vi "ziExample-Module-PIDAdvisor.vi"() -> ()   [LabVIEW 2009]
doc: "Control a Zurich instrument device via the LabOne Labview API. \nRequirements: Zurich Instruments HF2 +MF or UHFLI +MF \nPlease connect Signal input 1 and Signall Output 1.\nThis example shows how to configure a PID to regulate the output amplitude in order to achieve a constant input amplitude.\nThis example suggests a PID configuration via the PID advisor.\n\n© Zurich Instruments AG, www.zhinst.com"
uses:
  <instrlib>/Zurich Instruments LabOne/Public/ziTypeHandle.ctl
  <instrlib>/Zurich Instruments LabOne/Public/Modules/ziTypeModEnum.ctl
  <instrlib>/Zurich Instruments LabOne/Public/Modules/ziModSetValueBinary.vi
  <instrlib>/Zurich Instruments LabOne/Public/Configure/ziSetValueDouble.vi
  <instrlib>/Zurich Instruments LabOne/Public/Configure/ziSetValueDoubleArray.vi
  <instrlib>/Zurich Instruments LabOne/Public/Configure/ziGetValueString.vi
  <instrlib>/Zurich Instruments LabOne/Public/Modules/ziModSetValueDouble.vi
  <instrlib>/Zurich Instruments LabOne/Public/Modules/ziModSetValueDoubleArray.vi
  <instrlib>/Zurich Instruments LabOne/Public/Modules/ziModGetDoubleData.vi
  <instrlib>/Zurich Instruments LabOne/Public/Modules/ziModGetAdvisorData.vi
  <instrlib>/Zurich Instruments LabOne/Zurich Instruments LabOne.lvlib
panel:
  out "VALUE":dbl(graph)
  out "PID SHIFT":dbl(graph)
  out "demod/timeconstant":dbl
  out "Error Out":errorcluster
  out "Handle Out":T1 {"Handle" format="0x%08x"; "Conn" format="0x%08x"}
  in  "Calculate":bool
  in  "stop":bool
  out "PID ERROR":dbl(graph)
  in  "Address":string="DEV"
  in  "bw":dbl=100.0 caption="target BW (Hz)"
  in  "Mode":dbl(ring)=3.0 items=["P"=1.0, "I"=2.0, "PI"=3.0, "PID"=7.0, "PIDF"=15.0]
  out "i":dbl caption="I"
  out "p":dbl caption="P"
  out "dlimittimeconstant":dbl
  out "rate":dbl caption="Rate (Hz)"
  out "d":dbl caption="D"
  out "Step Response":cluster{"grid":dbl[], "r_avg":dbl[]}(graph)
  out "Bode Gain":cluster{"grid":dbl[], "r_avg":dbl[]}(graph)
  out "Bode Phase":cluster{"grid":dbl[], "r_avg":dbl[]}(graph)
  out "Selected Device":string
  in  "subscribepath":string="pidAdvisor/*" caption="Subscribe Path"
  # "ziExample-SweepModul.vi\nRequirements: UHFLI, HF2, MFLI +PID\nsee block diagram for VI description"
  # "Tested Devices:\n- UHFLI+PID \n- HF2+PID\n- MFLI+PID"
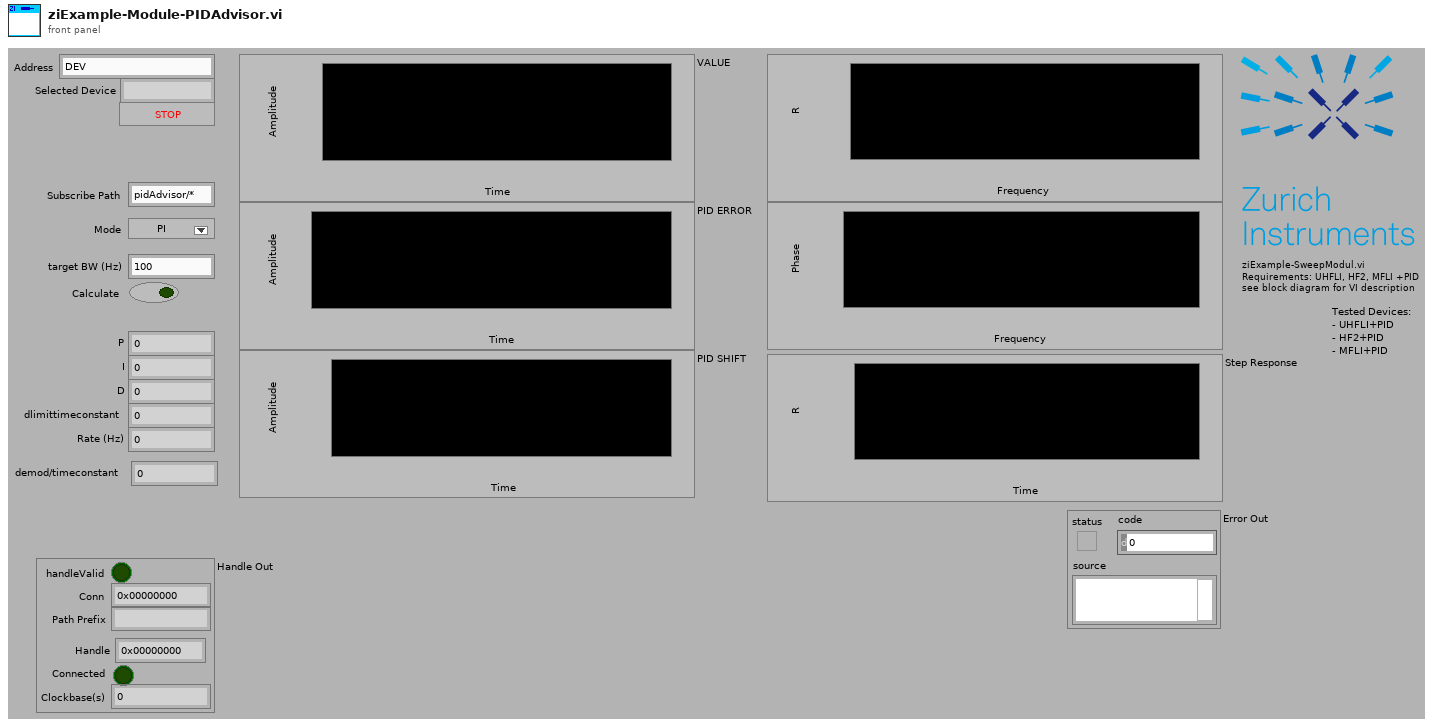
[diagram p1: front panel]
types:
  T1 = typedef "Zurich Instruments LabOne.lvlib/ziTypeHandle.ctl" = cluster{"handleValid":bool, "Conn":u64, "Path Prefix":string, "Handle":u64, "Connected":bool, "Clockbase(s)":dbl}
  T2 = typedef "Zurich Instruments LabOne.lvlib/ziTypeModEnum.ctl" = u16
  T3 = typedef "Zurich Instruments LabOne.lvlib/ziTypeModHandle.ctl" = cluster{"handleValid":bool, "Conn":u64, "ModHandle":u64, "moduleID":string, "Path Prefix":string}
  T4 = typedef "Zurich Instruments LabOne.lvlib/ziTypeModResults.ctl" = cluster{"PathArray":string[], "ValueType":T5, "NoOfResults":u64, "ziGenericHeader":T6[]}
  T5 = typedef "Zurich Instruments LabOne.lvlib/ziTypePollType.ctl" = enum16{"NONE", "DOUBLE_DATA", "INTEGER_DATA", "DEMOD_SAMPLE", "SCOPE_WAVE_HF2", "AUXIN_SAMPLE", "DIO_SAMPLE", "BYTE_ARRAY", "PWA_WAVE", "9", "10", "11", "12", "13", "14", "15", "TREE_CHANGE_DEPRI", "17", "ERROR", "19", "20", "21", "22", "23", "24", "25", "26", "27", "28", "29", "30", "31", "DOUBLE_DATA_TS", "INTEGER_DATA_TS", "34", "SCOPE_WAVE", "SCOPE_WAVE_EX", "37", "BYTE_ARRAY_TS", "39", "40", "41", "42", "43", "44", "45", "CNT_DATA", "47", "TREE_CHANGE", "49", "50", "51", "52", "53", "54", "55", "56", "57", "58", "59", "60", "61", "62", "63", "SWEEPER_DATA", "SPECTRUM_DATA", "ADVISOR_DATA", "VECTOR_DATA", "IMP_DATA"}
  T6 = typedef "Zurich Instruments LabOne.lvlib/ziTypeModGenericHeader.ctl" = cluster{"HeaderType":enum8{"HEADER_TYPE_NONE", "HEADER_TYPE_SWTRIGGER", "HEADER_TYPE_SWEEPER"}, "SampleFormat":u8, "SystemTime":timestamp, "CreatedTimeStamp":u64, "ChangedTimeStamp":u64, "Flags":u32, "ChunkSizeBytes":u64, "Name":string, "Status":u32, "GroupIndex":u32, "Color":u32, "ActiveRow":u32, "TriggerNumber":u64, "GridRows":u32, "GridCols":u32, "GridMode":u32, "GridOperation":u32, "GridDirection":u32, "GridRepetitions":u32, "GridColDelta":dbl, "GridColOffset":dbl, "GridRowDelta":dbl, "GridRowOffset":dbl, "Bandwidth":dbl, "Center":dbl, "Nenbw":dbl}
  T7 = typedef "Zurich Instruments LabOne.lvlib/ziTypeModAdvisorWave.ctl" = cluster{"timestamp":u64, "sampleCount":u64, "flags":u8, "sampleFormat":u8, "grid":dbl[], "x":dbl[], "y":dbl[]}
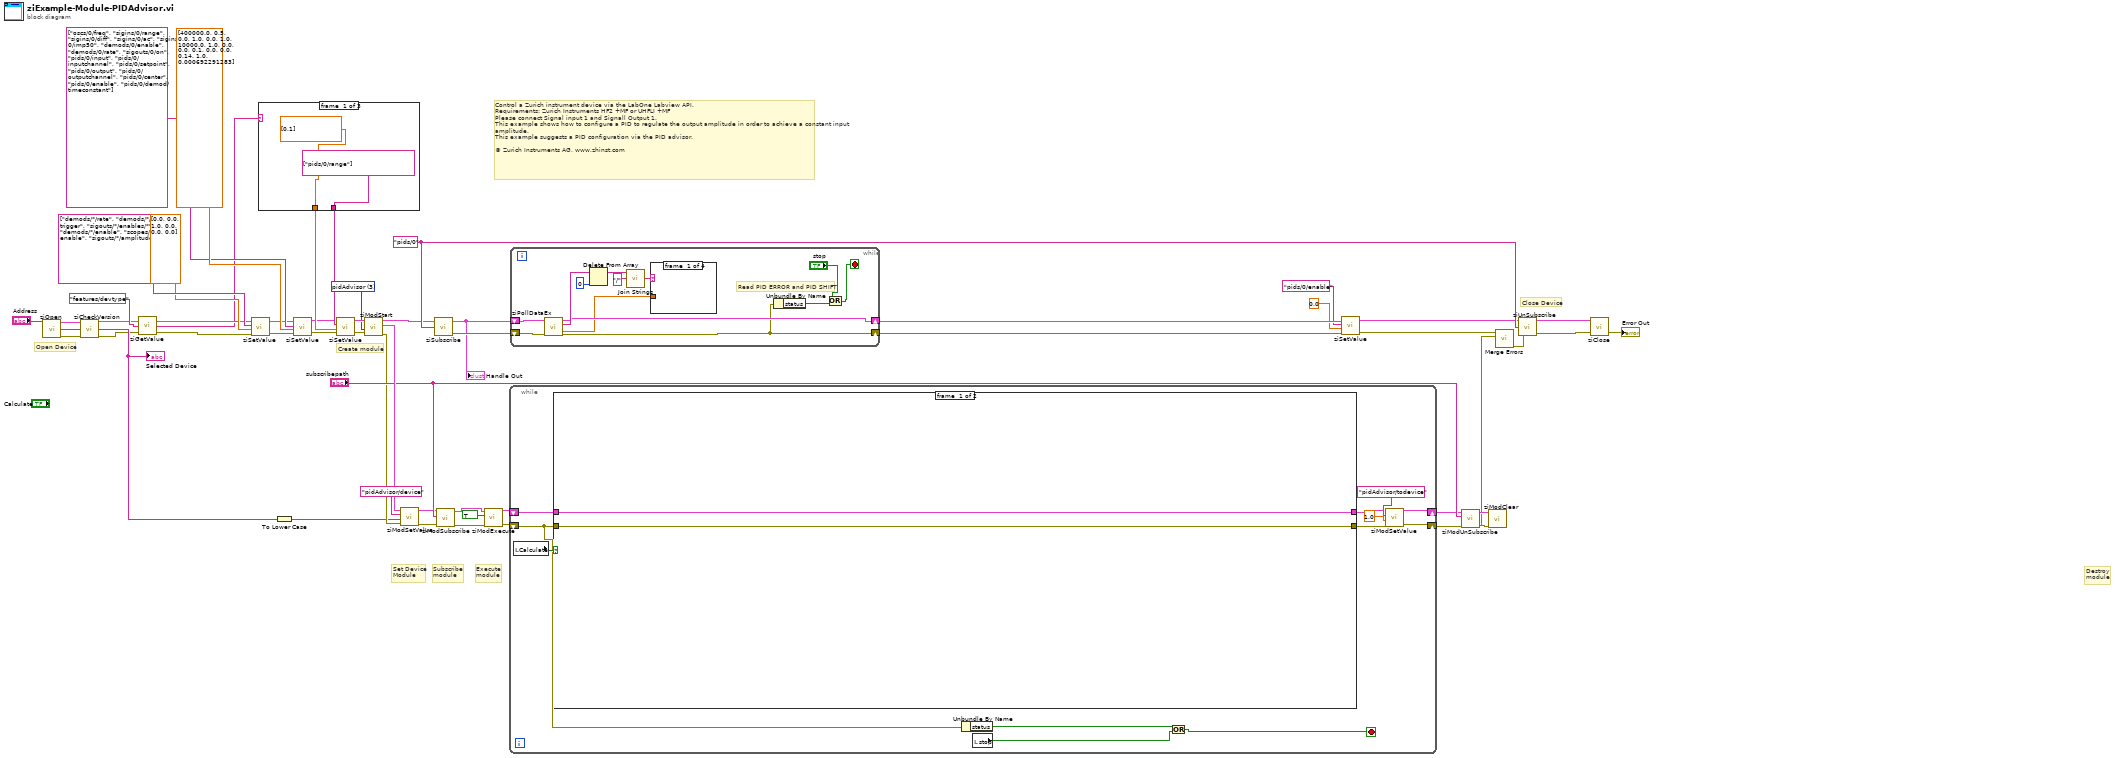
[diagram p0: block diagram]
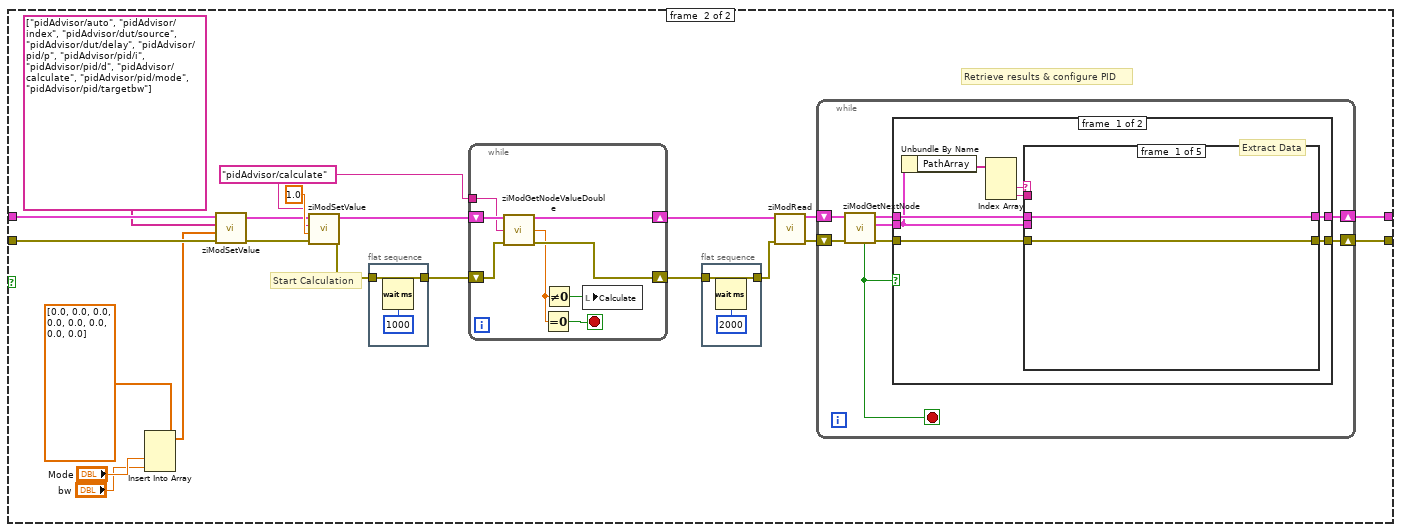
[diagram p2: hidden frame]
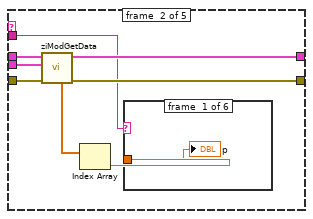
[diagram p3: hidden frame]
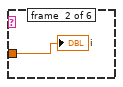
[diagram p4: hidden frame]
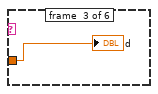
[diagram p5: hidden frame]
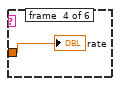
[diagram p6: hidden frame]
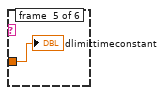
[diagram p7: hidden frame]
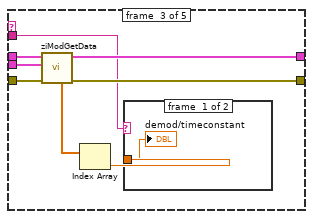
[diagram p9: hidden frame]
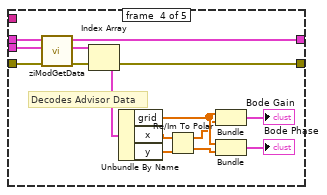
[diagram p11: hidden frame]
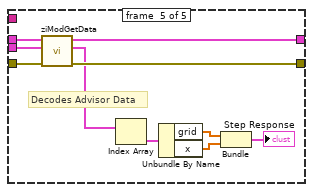
[diagram p12: hidden frame]
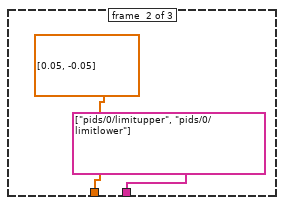
[diagram p14: hidden frame]
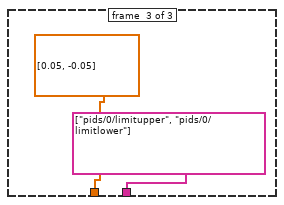
[diagram p15: hidden frame]
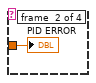
[diagram p16: hidden frame]
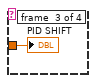
[diagram p17: hidden frame]
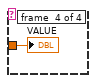
[diagram p18: hidden frame]
diagram:
  w1 = T2 3 items=["sweep", "scopeModule", "dataAcquisitionModule", "pidAdvisor", "awgModule", "impedanceModule", "multiDeviceSyncModule", "zoomFFT", "trigger", "deviceSettings", "record"] ("module Id")
  w29 = "pids/0" ("Path ()")
  # "Control a Zurich instrument device via the LabOne Labview API. \nRequirements: Zurich Instruments HF2 +MF or UHFLI +MF \nPlease connect Signal input 1 and Signall Output 1.\nThis example shows how to configure a PID to regulate the output amplitude in order to achieve a constant input amplitude.\nThis example suggests a PID configuration via the PID advisor.\n\n© Zurich Instruments AG, www.zhinst.com"
  # "Execute\nmodule"
  # "Set Device\nModule"
  # "Subscribe\nmodule"
  # "Destroy\nmodule"
  # "Create module"
  # "Close Device"
  # "Open Device"
  n1 = call <instrlib>:"ziOpen.vi"("Address"="Address") -> ("Error Out"=w2:errorcluster, "Selected Device"=w27:string, "HandleOut"=w5:T1)  [unwired: 1 in, 2 out]
  "Selected Device" <- w27
  n2 = call <instrlib>:"ziCheckVersion.vi"("Handle In"=w5, "Error In"=w2) -> ("Handle Out"=w4:T1, "Error Out"=w3:errorcluster)  [unwired: 11 in, 1 out]
  n3 = call-poly <instrlib>:"ziGetValue.vi"("error in"=w3, "Path"="features/devtype", "Handle In"=w4) -> ("error out"=w8:errorcluster, "Value"=w6:string, "Handle Out"=w9:T1)
  n4 = call-poly <instrlib>:"ziSetValue.vi"("Error In"=w8, "Values"=dbl[] [0.0, 0.0, 1.0, 0.0, 0.0, 0.0], "Paths"=string[] ["demods/*/rate", "demods/*/trigger", "sigouts/*/enables/*", "demods/*/enable", "scopes/*/enable", "sigouts/*/amplitudes/*"], "Handle In"=w9) -> ("Error Out"=w10:errorcluster, "Handle Out"=w11:T1)  [unwired: 1 in]
  n5 = case shown="\"MFIA\", \"MFLI\"" w6 {
    tunnel: [dbl[] [0.1] dbl[] [0.05, -0.05] dbl[] [0.05, -0.05]] -> w34
    tunnel: [string[] ["pids/0/range"] string[] ["pids/0/limitupper", "pids/0/limitlower"] string[] ["pids/0/limitupper", "pids/0/limitlower"]] -> w33
    frame #0 {
    }
    frame #1 {
    }
    frame #2 {
    }
  }
  n6 = To Lower Case(string=w27) -> (all lower case string=w26:string)
  n7 = call-poly <instrlib>:"ziSetValue.vi"("Error In"=w10, "Values"=dbl[] [400000.0, 0.5, 0.0, 1.0, 0.0, 1.0, 10000.0, 1.0, 0.0, 0.0, 0.1, 0.0, 0.0, 0.14, 1.0, 0.000692291283], "Paths"=string[] ["oscs/0/freq", "sigins/0/range", "sigins/0/diff", "sigins/0/ac", "sigins/0/imp50", "demods/0/enable", "demods/0/rate", "sigouts/0/on", "pids/0/input", "pids/0/inputchannel", "pids/0/setpoint", "pids/0/output", "pids/0/outputchannel", "pids/0/center", "pids/0/enable", "pids/0/demod/timeconstant"], "Handle In"=w11) -> ("Error Out"=w18:errorcluster, "Handle Out"=w19:T1)  [unwired: 1 in]
  n8 = call-poly <instrlib>:"ziSetValue.vi"("Error In"=w18, "Values"=w34, "Paths"=w33, "Handle In"=w19) -> ("Error Out"=w53:errorcluster, "Handle Out"=w54:T1)  [unwired: 1 in]
  n9 = call <instrlib>:"ziModStart.vi"("Error In"=w53, "module Id"=w1, "Handle In"=w54) -> ("Error Out"=w37:errorcluster, "ModHandle Out"=w50:T3, "Handle Out"=w7:T1)  [unwired: 6 in]
  n10 = call-poly <instrlib>:"ziModSetValue.vi"("Error In"=w37, "Data"=w26, "Path"="pidAdvisor/device", "ModHandle In"=w50) -> ("Error Out"=w41:errorcluster, "ModHandle Out"=w40:T3)  [unwired: 6 in]
  n11 = call <instrlib>:"ziSubscribe.vi"("Path ()"=w29, "Handle In"=w7) -> ("error out"=w51:errorcluster, "Handle Out"=w38:T1)  [unwired: 2 in]
  "Handle Out" <- w38
  n12 = call <instrlib>:"ziModSubscribe.vi"("Error In"=w41, "Path"="subscribepath", "ModHandle In"=w40) -> ("Error Out"=w48:errorcluster, "ModHandle Out"=w47:T3)  [unwired: 6 in]
  n13 = call <instrlib>:"ziModExecute.vi"("Error In"=w48, "Modal (F)"=TRUE ("Modal"), "ziModHandle In"=w47) -> ("Error Out"=w49:errorcluster, "ziModHandle Out"=w39:T3)  [unwired: 5 in, 1 out]
  n14 = while {
    shift-right: [w67] -> w13
    shift-left: w39 -> [w72]
    shift-right: [w66] -> w12
    shift-left: w49 -> [w64]
    stop <- w61 stop-if-true
    n15 = local read "Calculate"() -> (w71:bool)
    n16 = case shown="True" w71 {
      tunnel: w72 -> [w73 w89]
      tunnel: w64 -> [w74 w90]
      tunnel: [w74 w82] -> w65
      tunnel: [w73 w83] -> w68
      frame #0 {
      }
      frame #1 {
        w76 = "pidAdvisor/calculate" ("Path")
        # "Extract Data"
        # "Retrieve results & configure PID"
        # "Start Calculation"
        n17 = Insert Into Array(array=dbl[] [0.0, 0.0, 0.0, 0.0, 0.0, 0.0, 0.0, 0.0], new element #1="Mode", new element #2="bw") -> (w77:dbl[])  [unwired: 1 in]
        n18 = call-poly <instrlib>:"ziModSetValue.vi"("Error In"=w90, "Values"=w77, "Paths"=string[] ["pidAdvisor/auto", "pidAdvisor/index", "pidAdvisor/dut/source", "pidAdvisor/dut/delay", "pidAdvisor/pid/p", "pidAdvisor/pid/i", "pidAdvisor/pid/d", "pidAdvisor/calculate", "pidAdvisor/pid/mode", "pidAdvisor/pid/targetbw"], "ModHandle In"=w89) -> ("Error Out"=w75:errorcluster, "ModHandle Out"=w78:T3)  [unwired: 6 in]
        n19 = call-poly <instrlib>:"ziModSetValue.vi"("Error In"=w75, "Value"=1.0, "Path"=w76, "ModHandle In"=w78) -> ("Error Out"=w88:errorcluster, "ModHandle Out"=w93:T3)  [unwired: 6 in]
        n20 = flat-sequence {
          tunnel: [w99] -> w87
          tunnel: w88 -> [w99]
          frame #0 {
            n21 = Wait (ms)(milliseconds to wait=u32 1000) -> ()  [unwired: 1 out]
          }
        }
        n22 = while {
          shift-right: [w169] -> w94
          shift-left: w93 -> [w172]
          shift-right: [w170] -> w85
          shift-left: w87 -> [w173]
          tunnel: w76 -> [w171]
          stop <- w168 stop-if-true
          n23 = call <instrlib>:"ziModGetNodeValueDouble.vi"("ModHandle In"=w172, "Path"=w171, "error in"=w173) -> ("ModHandle Out"=w169:T3, "Value"=w166:dbl, "error out"=w170:errorcluster)  [unwired: 10 in]
          n24 = Equal To 0?(x=w166) -> (x = 0?=w168:bool)
          n25 = Not Equal To 0?(x=w166) -> (x != 0?=w167:bool)
          n26 = local write "Calculate"(w167) -> ()
        }
        n27 = flat-sequence {
          tunnel: w85 -> [w96]
          tunnel: [w96] -> w84
          frame #0 {
            n28 = Wait (ms)(milliseconds to wait=u32 2000) -> ()  [unwired: 1 out]
          }
        }
        n29 = call <instrlib>:"ziModRead.vi"("error in"=w84, "ziModHandle In"=w94) -> ("error out"=w91:errorcluster, "ziModHandle Out"=w92:T3)  [unwired: 8 in]
        n30 = while {
          shift-right: [w101] -> w83
          shift-left: w92 -> [w106]
          shift-right: [w100] -> w82
          shift-left: w91 -> [w107]
          stop <- w102 stop-if-true
          n31 = call <instrlib>:"ziModGetNextNode.vi"("Error In"=w107, "ModHandle In"=w106) -> ("Error Out"=w104:errorcluster, "ModResults"=w103:T4, "ModHandle Out"=w105:T3, "NoData"=w102:bool)  [unwired: 6 in]
          n32 = case shown="False" w102 {
            tunnel: w105 -> [w115 w165]
            tunnel: w104 -> [w114 w164]
            tunnel: w103 -> [w111 _]
            tunnel: [w113 w165] -> w101
            tunnel: [w112 w164] -> w100
            frame #0 {
              n33 = Unbundle By Name(w111) -> ("PathArray"=w110:string[])
              n34 = Index Array(array=w110) -> (element #2=w108:string, element #3=w109:string)  [unwired: 3 in, 1 out]
              n35 = case shown="Default" w108 {
                tunnel: w115 -> [w117 w125 w138 w152 w162]
                tunnel: w111 -> [_ w124 w137 w153 w163]
                tunnel: w114 -> [w116 w123 w136 w151 w161]
                tunnel: [w116 w120 w133 w150 w160] -> w112
                tunnel: [w117 w122 w135 w149 w159] -> w113
                tunnel: w109 -> [_ w119 w132 _ _]
                frame #0 {
                }
                frame #1 {
                  n36 = call-poly <instrlib>:"ziModGetData.vi"("Error In"=w123, "ModResults"=w124, "ModHandle In"=w125) -> ("Error Out"=w120:errorcluster, "ModHandle Out"=w122:T3, "Value"=w118:dbl[])  [unwired: 4 in, 2 out]
                  n37 = Index Array(array=w118) -> (element=w121:dbl)  [unwired: 1 in]
                  n38 = case shown="\"d\"" w119 {
                    tunnel: w121 -> [w126 w127 w128 w129 w130 _]
                    frame #0 {
                      "p" <- w126
                    }
                    frame #1 {
                      "i" <- w127
                    }
                    frame #2 {
                      "d" <- w128
                    }
                    frame #3 {
                      "rate" <- w129
                    }
                    frame #4 {
                      "dlimittimeconstant" <- w130
                    }
                    frame #5 {
                    }
                  }
                }
                frame #2 {
                  n39 = call-poly <instrlib>:"ziModGetData.vi"("Error In"=w136, "ModResults"=w137, "ModHandle In"=w138) -> ("Error Out"=w133:errorcluster, "ModHandle Out"=w135:T3, "Value"=w131:dbl[])  [unwired: 4 in, 2 out]
                  n40 = Index Array(array=w131) -> (element=w134:dbl)  [unwired: 1 in]
                  n41 = case shown="\"timeconstant\"" w132 {
                    tunnel: w134 -> [w139 _]
                    frame #0 {
                      "demod/timeconstant" <- w139
                    }
                    frame #1 {
                    }
                  }
                }
                frame #3 {
                  # "Decodes Advisor Data"
                  n42 = call-poly <instrlib>:"ziModGetData.vi"("Error In"=w151, "ModResults"=w153, "ModHandle In"=w152) -> ("Error Out"=w150:errorcluster, "AdvisorData Out"=w147:T7[], "ModHandle Out"=w149:T3)  [unwired: 6 in]
                  n43 = Index Array(array=w147) -> (element=w148:T7)  [unwired: 1 in]
                  n44 = Unbundle By Name(w148) -> ("grid"=w144:dbl[], "x"=w140:dbl[], "y"=w141:dbl[])
                  n45 = Re/Im To Polar(2:w141, 3:w140) -> (0:w142:dbl[], 1:w143:dbl[])
                  n46 = Bundle("grid"=w144, w143) -> (→"Bode Gain":cluster{"grid":dbl[], dbl[]})  [unwired: 1 in]
                  n47 = Bundle("grid"=w144, w142) -> (→"Bode Phase":cluster{"grid":dbl[], dbl[]})  [unwired: 1 in]
                }
                frame #4 {
                  # "Decodes Advisor Data"
                  n48 = call-poly <instrlib>:"ziModGetData.vi"("Error In"=w161, "ModResults"=w163, "ModHandle In"=w162) -> ("Error Out"=w160:errorcluster, "AdvisorData Out"=w157:T7[], "ModHandle Out"=w159:T3)  [unwired: 6 in]
                  n49 = Index Array(array=w157) -> (element=w158:T7)  [unwired: 1 in]
                  n50 = Unbundle By Name(w158) -> ("grid"=w156:dbl[], "x"=w155:dbl[])
                  n51 = Bundle("grid"=w156, "x"=w155) -> (→"Step Response":cluster{"grid":dbl[], "x":dbl[]})  [unwired: 1 in]
                }
              }
            }
            frame #1 {
              (unwired) FALSE
            }
          }
        }
      }
    }
    n52 = Unbundle By Name(w64) -> ("status"=w63:bool)
    n53 = local read "stop"() -> (w62:bool)
    n54 = Or(x=w63, y=w62) -> (x .or. y?=w61:bool)
    n55 = call-poly <instrlib>:"ziModSetValue.vi"("Error In"=w65, "Value"=1.0, "Path"="pidAdvisor/todevice", "ModHandle In"=w68) -> ("Error Out"=w66:errorcluster, "ModHandle Out"=w67:T3)  [unwired: 6 in]
  }
  n56 = while {
    shift-right: [w179] -> w24
    shift-left: w38 -> [w186]
    shift-right: [w177] -> w25
    shift-left: w51 -> [w185]
    stop <- w174 stop-if-true
    # "Read PID ERROR and PID SHIFT"
    n57 = call <instrlib>:"ziPollDataEx.vi"("error in"=w185, "Handle In"=w186) -> ("error out"=w177:errorcluster, "PathArray"=w183:string[], "Handle Out"=w179:T1, "Value Double"=w178:dbl)  [unwired: 2 in, 4 out]
    n58 = Delete From Array(array=w183, index=0) -> (array with subset deleted=w182:string[])  [unwired: 1 in, 1 out]
    n59 = call <vilib>:"Join Strings.vi"("Separator (,)"="/" ("delimiter (Tab)"), "Strings In"=w182) -> ("String"=w180:string)  [unwired: 1 in]
    n60 = case shown="\"PIDS/0/STREAM/VALUE\", \"PIDS/0/VALUE\"" w180 {
      tunnel: w178 -> [_ w187 w188 w189]
      frame #0 {
      }
      frame #1 {
        "PID ERROR" <- w187
      }
      frame #2 {
        "PID SHIFT" <- w188
      }
      frame #3 {
        "VALUE" <- w189
      }
    }
    n61 = Unbundle By Name(w177) -> ("status"=w176:bool)
    n62 = Or(x="stop", y=w176) -> (x .or. y?=w174:bool)
  }
  n63 = call-poly <instrlib>:"ziSetValue.vi"("Error In"=w25, "Value"=0.0, "Path"="pids/0/enable", "Handle In"=w24) -> ("Error Out"=w16:errorcluster, "Handle Out"=w23:T1)  [unwired: 1 in]
  n64 = call <instrlib>:"ziModUnSubscribe.vi"("Error In"=w12, "Path (\"/\")"="subscribepath", "ModHandle In"=w13) -> ("Error Out"=w42:errorcluster, "ModHandle Out"=w43:T3)  [unwired: 7 in]
  n65 = call <instrlib>:"ziModClear.vi"("Error In"=w42, "ziModHandle In"=w43) -> ("Error Out"=w17:errorcluster)  [unwired: 7 in, 1 out]
  n66 = call <vilib>:"Merge Errors.vi"("error in 2 (no error)"=w17, "error in 1 (no error)"=w16) -> ("error out"=w14:errorcluster)  [unwired: 5 in]
  n67 = call <instrlib>:"ziUnSubscribe.vi"("error in"=w14, "Path (\"/\")"=w29, "Handle in"=w23) -> ("error out"=w15:errorcluster, "Handle out"=w28:T1)  [unwired: 1 in]
  n68 = call <instrlib>:"ziClose.vi"("Error In"=w15, "Handle In"=w28) -> ("Error Out"=→"Error Out":errorcluster)  [unwired: 2 in, 1 out]
